vi "Format Error.vi"(7 "subsource (needed for inlined methods)":string, 8 "error in (no error)":errorcluster, 9 "Additional source description":string, 10 "error message":string, 11 "error code":T1) -> (0 "error out":errorcluster)   [LabVIEW 2013, in "PQ Connection.lvclass"]
uses:
  PQ Connection.lvclass
  Connection Status.ctl
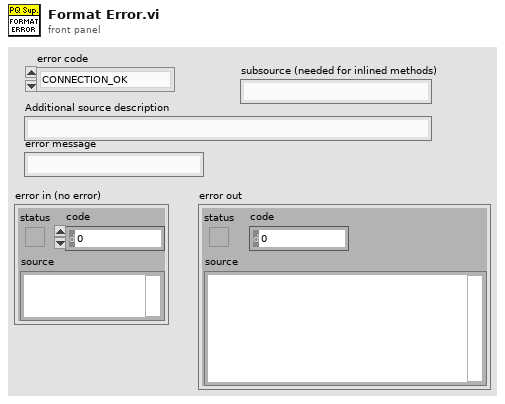
[diagram p1: front panel]
types:
  T1 = typedef "PQ Connection.lvclass/Connection Status.ctl" = enum32{"CONNECTION_OK", "CONNECTION_BAD", "CONNECTION_STARTED", "CONNECTION_MADE", "CONNECTION_AWAITING_RESPONSE", "CONNECTION_AUTH_OK", "CONNECTION_SETENV", "CONNECTION_SSL_STARTUP", "CONNECTION_NEEDED"}
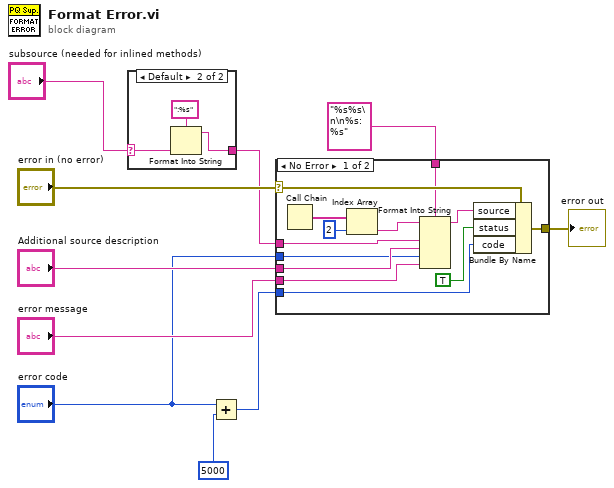
[diagram p0: block diagram]
diagram:
  n1 = case shown="Default" "subsource (needed for inlined methods)" {
    selector: "subsource (needed for inlined methods)" -> [w11 w14]
    tunnel: [w11 w12] -> w2
    frame "" {
    }
    frame Default {
      n2 = Format Into String(format string=":%s", w14) -> (resulting string=w12:string)  [unwired: 2 in, 1 out]
    }
  }
  n3 = Add(x="error code", y=5000) -> (x+y=w7:u32)
  n4 = case shown="No Error" "error in (no error)" {
    selector: "error in (no error)" -> [w24 w28]
    tunnel: "error message" -> [w19 _]
    tunnel: w7 -> [w23 _]
    tunnel: [w25 w28] -> w8
    tunnel: "Additional source description" -> [w20 _]
    tunnel: "%s%s\n\n%s: %s" ("format string") -> [w18 _]
    tunnel: w2 -> [w16 _]
    tunnel: "error code" -> [w15 _]
    frame No Error {
      n5 = Call Chain() -> (call chain=w21:string[])
      n6 = Index Array(array=w21, index=2) -> (element=w17:string)
      n7 = Format Into String(format string=w18, initial string=w17, w16, w20, w15, w19) -> (resulting string=w27:string)  [unwired: 1 in, 1 out]
      n8 = Bundle By Name(cluster=w24, "source"=w27, "status"=TRUE, "code"=w23) -> (w25:errorcluster)
    }
    frame Error {
    }
  }
  "error out" <- w8
